vi "Read.vi"(8 "error in (no error)":errorcluster, 11 "Simulate in":refnum<class "Simulated DMM.lvclass">) -> (0 "error out":errorcluster, 1 "String":string, 2 "Measurement":dbl format="%.5f", 3 "Simulate out":refnum<class "Simulated DMM.lvclass">)   [LabVIEW 2012, in "Simulated DMM.lvclass"]
uses:
  Simulated DMM.lvclass
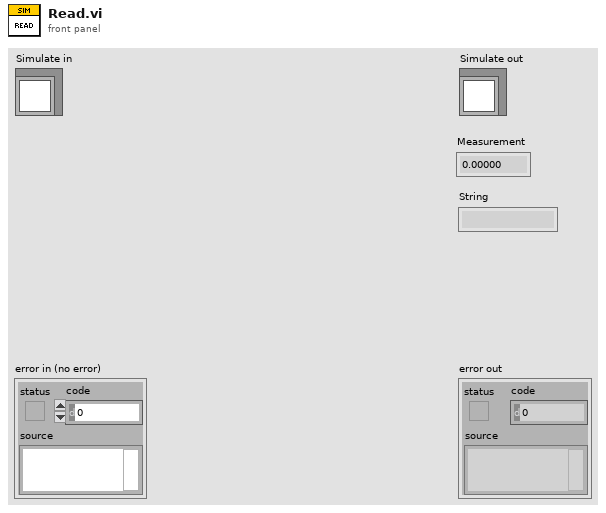
[diagram p1: front panel]
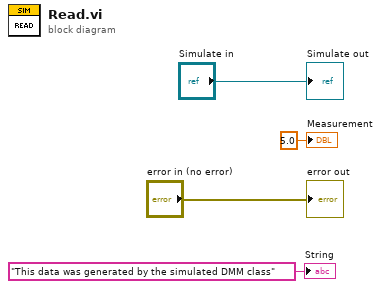
[diagram p0: block diagram]
diagram:
  "error out" <- "error in (no error)"
  "Simulate out" <- "Simulate in"
  "Measurement" <- 5.0 ("Measurement")
  "String" <- "This data was generated by the simulated DMM class" ("String")
